vi "Configure Burst Operation.vi"(4 "Burst Period (0.01 s)":dbl=0.01 min=1e-06 max=500.0 format="%#.6g", 5 "Gate Polarity (Normal)":enum16{"Normal", "Inverted"}(ring), 6 "Burst Count (1)":i32=1 min=0 max=50000, 7 "Enable Burst Operation (Enable)":bool=TRUE, 8 "error in (no error)":errorcluster, 9 "Burst Phase  (0 Degrees)":i32 min=-360 max=360, 10 "Burst Mode (Triggered)":enum16{"Triggered", "Gated"}(ring), 11 "VISA resource name":refnum<visa-resource-name>) -> (0 "error out":errorcluster, 3 "VISA resource name out":refnum<visa-resource-name>)   [LabVIEW 2017, in "Keithley 3390.lvlib"]
doc: "Configures and enables burst operation. In burst mode the function generator outputs the waveform for a finite number of cycles upon the reception of a trigger rather than continuously forever."
uses:
  Keithley 3390.lvlib
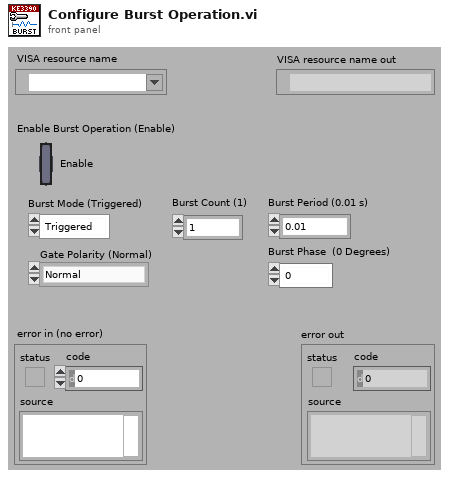
[diagram p1: front panel]
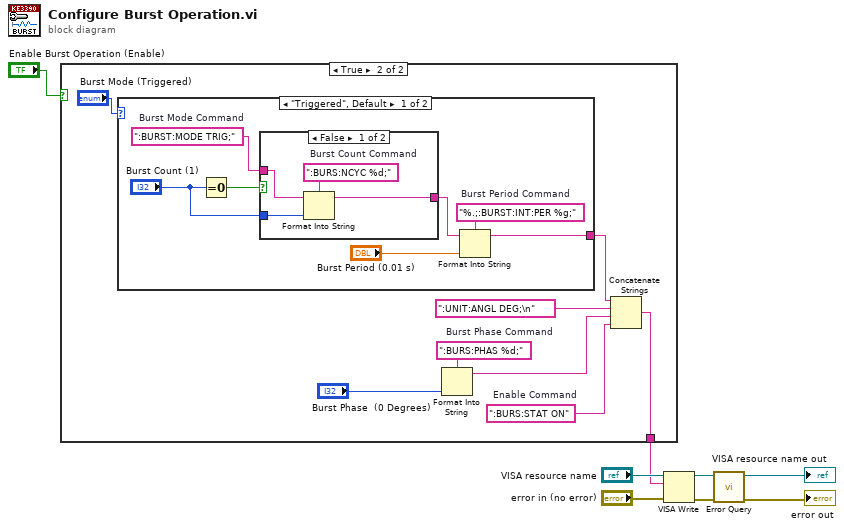
[diagram p0: block diagram]
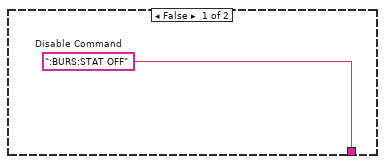
[diagram p2: hidden frame]
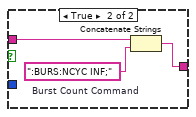
[diagram p3: hidden frame]
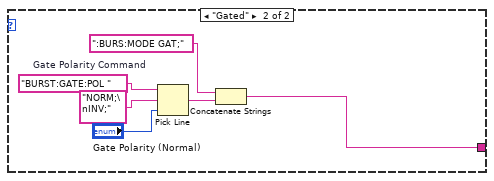
[diagram p4: hidden frame]
diagram:
  n1 = case shown="True" "Enable Burst Operation (Enable)" {
    tunnel: [w9 w10] -> w1
    frame False {
      w9 = ":BURS:STAT OFF"  # Disable Command
    }
    frame True {
      w16 = ":BURS:PHAS %d;"  # Burst Phase Command
      w11 = ":BURS:STAT ON"  # Enable Command
      n2 = case shown="\"Triggered\", Default" "Burst Mode (Triggered)" {
        tunnel: [w21 w32] -> w14
        frame "Triggered", Default {
          w24 = "%.;:BURST:INT:PER %g;"  # Burst Period Command
          w18 = ":BURST:MODE TRIG;"  # Burst Mode Command
          n3 = Equal To 0?(x="Burst Count (1)") -> (x = 0?=w20:bool)
          n4 = case shown="False" w20 {
            tunnel: [w27 w30] -> w22
            tunnel: "Burst Count (1)" -> [w26 _]
            tunnel: w18 -> [w25 w31]
            frame False {
              w28 = ":BURS:NCYC %d;"  # Burst Count Command
              n5 = Format Into String(format string=w28, initial string=w25, w26) -> (resulting string=w27:string)  [unwired: 1 in, 1 out]
            }
            frame True {
              w29 = ":BURS:NCYC INF;"  # Burst Count Command
              n6 = Concatenate Strings(w31, w29) -> (w30:string)
            }
          }
          n7 = Format Into String(format string=w24, initial string=w22, "Burst Period (0.01 s)") -> (resulting string=w21:string)  [unwired: 1 in, 1 out]
        }
        frame "Gated" {
          w35 = "BURST:GATE:POL "  # Gate Polarity Command
          n8 = Pick Line(string ("")=w35, multi-line string="NORM;\nINV;", line index="Gate Polarity (Normal)") -> (output string=w33:string)
          n9 = Concatenate Strings(":BURS:MODE GAT;", w33) -> (w32:string)
        }
      }
      n10 = Format Into String(format string=w16, "Burst Phase  (0 Degrees)") -> (resulting string=w12:string)  [unwired: 2 in, 1 out]
      n11 = Concatenate Strings(w14, ":UNIT:ANGL DEG;\n", w12, w11) -> (w10:string)
    }
  }
  n12 = VISA Write(VISA resource name="VISA resource name", write buffer=w1, error in (no error)="error in (no error)") -> (VISA resource name out=w6:refnum<visa-resource-name>, error out=w4:errorcluster)  [unwired: 1 out]
  n13 = call "Error Query.vi"("error in (no error)"=w4, "VISA resource name"=w6) -> ("error out"=→"error out":errorcluster, "VISA resource name out"=→"VISA resource name out":refnum<visa-resource-name>)  [unwired: 6 in, 2 out]
